vi "ConfigureHallsensorSensorType.vi"(4 "error in (no error)":errorcluster, 5 "SensorType":u16(ring)=3 items=["Unknown sensor", "Incremental encoder with index (3-channel)", "Incremental encoder without index (2-channel)", "Hall sensors", "SSI encoder binary coded", "SSI encoder grey coded"], 6 "hallsensor configuration":cluster{"invertedPolarity":i32}, 7 "axis in":cluster{"keyHandle":u32, "nodeId":u16}={"keyHandle"=0, "nodeId"=1}) -> (0 "error out":errorcluster, 3 "axis out":cluster{"keyHandle":u32, "nodeId":u16}={"keyHandle"=0, "nodeId"=1})   [LabVIEW 2018]
doc: "<B>ConfigureHallsensorSensorType</B> writes the value for sensor type 'hallsensor' to the device. Parameters from the sensor type can be set."
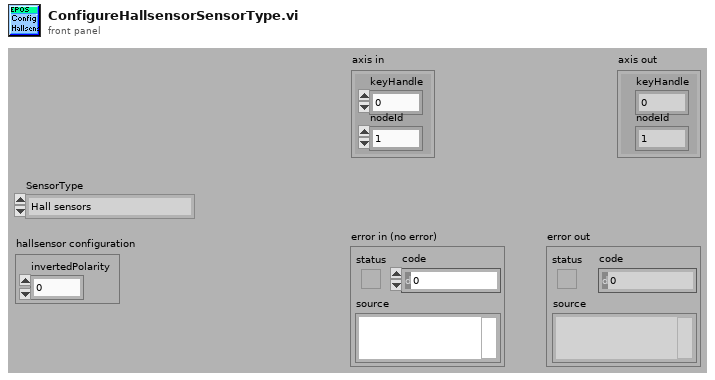
[diagram p1: front panel]
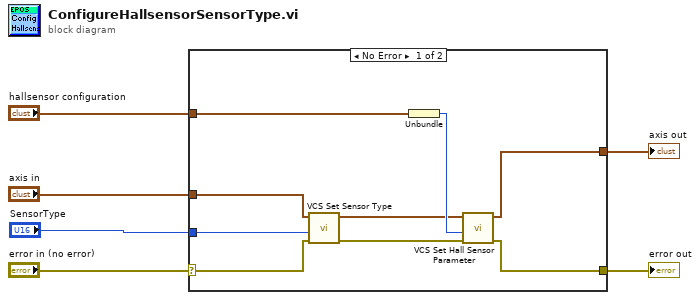
[diagram p0: block diagram]
diagram:
  n1 = case shown="No Error" "error in (no error)" {
    selector: "error in (no error)" -> [w14 w17]
    tunnel: [w8 w17] -> w5
    tunnel: [w9 w16] -> w4
    tunnel: "axis in" -> [w15 w16]
    tunnel: "SensorType" -> [w13 _]
    tunnel: "hallsensor configuration" -> [w12 _]
    frame No Error {
      n2 = call "VCS Set Sensor Type.vi"("error in (no error)"=w14, "SensorType"=w13, "axis in"=w15) -> ("error out"=w7:errorcluster, "axis out"=w10:cluster{"keyHandle":u32, "nodeId":u16})  [unwired: 7 in]
      n3 = Unbundle(w12) -> ("invertedPolarity"=w11:i32)
      n4 = call "VCS Set Hall Sensor Parameter.vi"("error in (no error)"=w7, "invertedPolarity"=w11, "axis in"=w10) -> ("error out"=w8:errorcluster, "axis out"=w9:cluster{"keyHandle":u32, "nodeId":u16})  [unwired: 7 in]
    }
    frame Error {
    }
  }
  "error out" <- w5
  "axis out" <- w4
